vi "_Validate Lens Property.vi"(6 "Lens Property In":T8={"Scan Type"=0, "Unit"=TRUE, "Count1"=1.0, "Count2"=1.0, "Time1"=1.0, "Time2"=1.0, "Scans"=1, "Step Size"=1.0, "Row Numer"=0} {"Scan Type" items=["Single", "Dual", "Ramp"]}, 8 "Method In":T1={"Lenses"=[], "Mass Ranges"=[], "Acquire"=FALSE, "MCA"=FALSE, "Q1DC EN"=FALSE, "Q1 POL"=FALSE, "Q3 POL"=FALSE, "Q1 RF  EN"=FALSE, "Averaging"=FALSE, "Log Scale"=FALSE, "CPS"=FALSE, "Unit"=FALSE, "Data Path"=path "", "Run Mode"=enum."MRM (Q1/Q2)", "Fixed Mass (amu)"=1.0, "Q3DC EN"=FALSE, "Q3 RF  EN"=FALSE, "Negative"=FALSE} {"Mass Ranges"."Res" items=["High/High", "Medium/Medium", "Low/Low", "High/Medium", "High/Low", "Medium/High", "Medium/Low", "Low/High", "Low/Medium"]}) -> (0 "Lens Table":string[][](table), 1 "Lens Property Out":T7={"Scan Type"=0, "Unit"=TRUE, "Count1"=1.0, "Count2"=1.0, "Time1"=1.0, "Time2"=1.0, "Scans"=1, "Step Size"=1.0, "Start DAC"=1, "Ramp Time (ms)"=1} {"Scan Type" items=["Single", "Dual", "Ramp"]}, 3 "Method Out":T1={"Lenses"=[], "Mass Ranges"=[], "Acquire"=FALSE, "MCA"=FALSE, "Q1DC EN"=FALSE, "Q1 POL"=FALSE, "Q3 POL"=FALSE, "Q1 RF  EN"=FALSE, "Averaging"=FALSE, "Log Scale"=FALSE, "CPS"=FALSE, "Unit"=FALSE, "Data Path"=path "", "Run Mode"=enum."MRM (Q1/Q2)", "Fixed Mass (amu)"=1.0, "Q3DC EN"=FALSE, "Q3 RF  EN"=FALSE, "Negative"=FALSE} {"Mass Ranges"."Res" items=["High/High", "Medium/Medium", "Low/Low", "High/Medium", "High/Low", "Medium/High", "Medium/Low", "Low/High", "Low/Medium"]})   [LabVIEW 2012]
uses:
  Type/_GUI Method.ctl
  Type/_Lens Property.ctl
  Type/_Mass Range Property.ctl
  Type/_Mass Range Parameters.ctl
  Type/_RT Res Type.ctl
  Type/_Run Mode.ctl
  _Global Configuration.vi
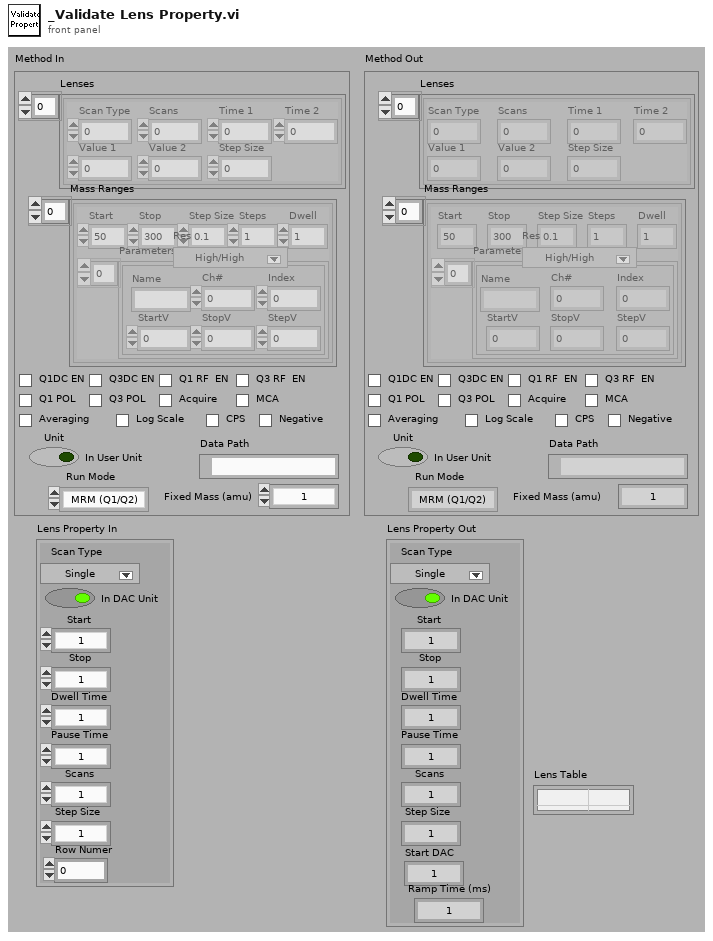
[diagram p1: front panel]
types:
  T1 = typedef "_GUI Method.ctl" = cluster{"Lenses":T2[], "Mass Ranges":T3[], "Acquire":bool, "MCA":bool, "Q1DC EN":bool, "Q1 POL":bool, "Q3 POL":bool, "Q1 RF  EN":bool, "Averaging":bool, "Log Scale":bool, "CPS":bool, "Unit":bool, "Data Path":path, "Run Mode":T6, "Fixed Mass (amu)":dbl, "Q3DC EN":bool, "Q3 RF  EN":bool, "Negative":bool}
  T2 = typedef "_Lens Property.ctl" = cluster{"Scan Type":u8, "Scans":i32, "Time 1":dbl, "Time 2":dbl, "Value 1":dbl, "Value 2":dbl, "Step Size":dbl}
  T3 = typedef "_Mass Range Property.ctl" = cluster{"Start":dbl, "Stop":dbl, "Step Size":dbl, "Steps":i32, "Dwell":dbl, "Parameters":T4[], "Res":T5}
  T4 = typedef "_Mass Range Parameters.ctl" = cluster{"Name":string, "Ch#":u8, "StartV":dbl, "StopV":dbl, "StepV":dbl, "Index":u8}
  T5 = typedef "_RT Res Type.ctl" = u16
  T6 = typedef "_Run Mode.ctl" = enum16{"MRM (Q1/Q2)", "Q1 Scan", "Q1 SRM", "Q2 Scan", "Q2 SRM", "Product Scan", "Precursor Scan", "Neutral Loss", "Neutral Gain"}
  T7 = cluster{"Scan Type":u8, "Unit":bool, "Count1":dbl, "Count2":dbl, "Time1":dbl, "Time2":dbl, "Scans":i32, "Step Size":dbl, "Start DAC":i32, "Ramp Time (ms)":i32}
  T8 = cluster{"Scan Type":u8, "Unit":bool, "Count1":dbl, "Count2":dbl, "Time1":dbl, "Time2":dbl, "Scans":i32, "Step Size":dbl, "Row Numer":i32}
  T9 = typedef "_RT Instrument 2.ctl" = cluster{"Table":T10[], "Instrument":string[]}
  T10 = typedef "_RT Configuration 2.ctl" = cluster{"Name":string, "Ch#":u8, "Min":dbl, "Max":dbl, "Def+":dbl, "Def-":dbl, "Offset":dbl, "Slope":dbl, "Type":u8, "Description":string, "SettleT":dbl}
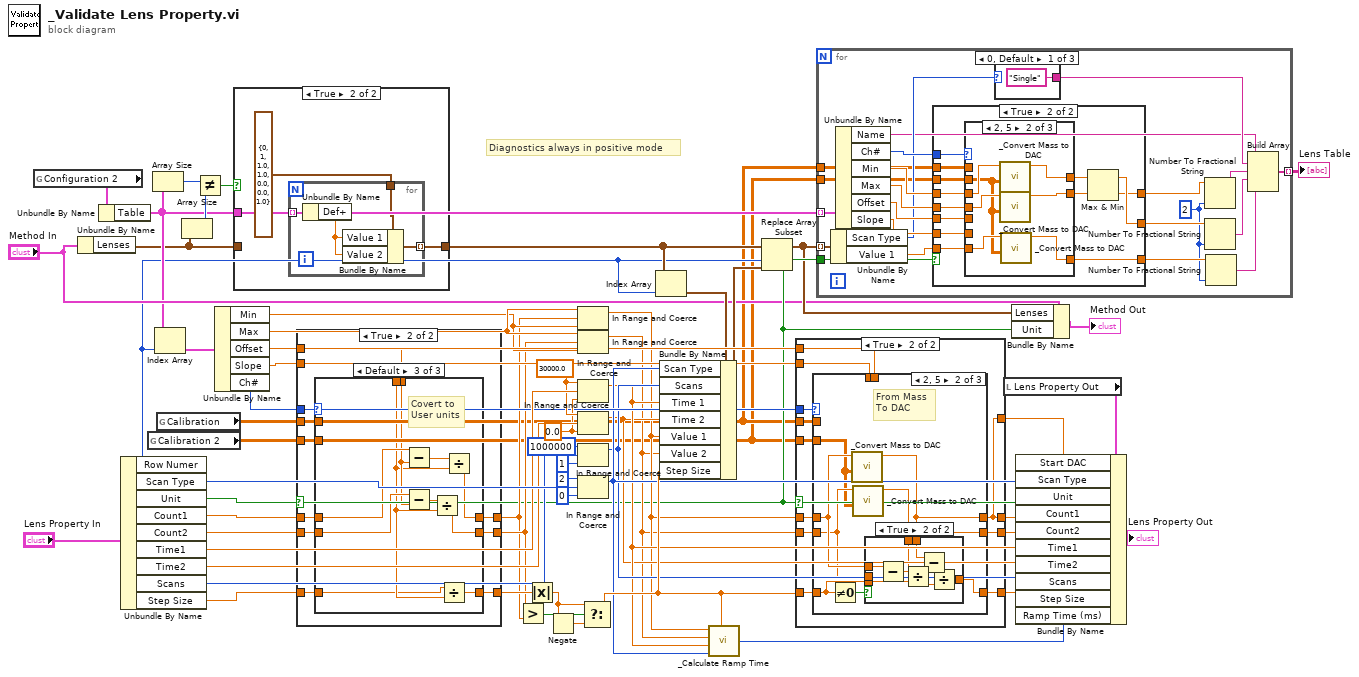
[diagram p0: block diagram]
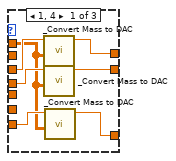
[diagram p4: hidden frame]
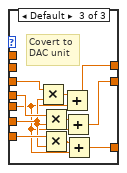
[diagram p5: hidden frame]
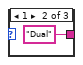
[diagram p6: hidden frame]
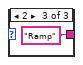
[diagram p7: hidden frame]
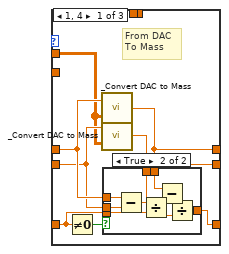
[diagram p9: hidden frame]
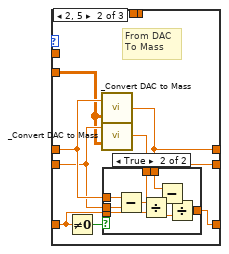
[diagram p11: hidden frame]
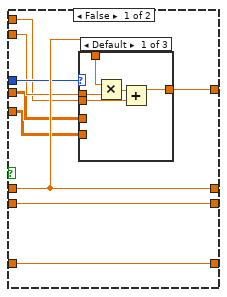
[diagram p13: hidden frame]
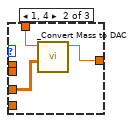
[diagram p14: hidden frame]
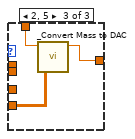
[diagram p15: hidden frame]
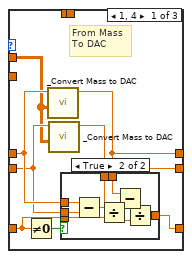
[diagram p16: hidden frame]
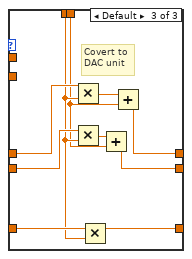
[diagram p19: hidden frame]
diagram:
  w41 = 0.0 ("lower limit")
  w43 = 30000.0 ("upper limit")
  # "Diagnostics always in positive mode"
  n1 = global read "_Global Configuration.vi" "Configuration 2"() -> (w26:T9)
  n2 = Unbundle By Name("Method In") -> ("Lenses"=w8:T2[])
  n3 = Unbundle By Name(w26) -> ("Table"=w9:T10[])
  n4 = Unbundle By Name("Lens Property In") -> ("Row Numer"=w6:i32, "Scan Type"=w57:u8, "Unit"=w16:bool, "Count1"=w56:dbl, "Count2"=w55:dbl, "Time1"=w54:dbl, "Time2"=w53:dbl, "Scans"=w52:i32, "Step Size"=w51:dbl)
  n5 = global read "_Global Configuration.vi" "Calibration 2"() -> (w1:dbl[][])
  n6 = Array Size(array=w9) -> (size(s)=w12:i32)
  n7 = Index Array(array=w9, index=w6) -> (element=w25:T10)
  n8 = global read "_Global Configuration.vi" "Calibration"() -> (w2:dbl[][])
  n9 = Array Size(array=w8) -> (size(s)=w13:i32)
  n10 = Not Equal?(x=w12, y=w13) -> (x != y?=w11:bool)
  n11 = Unbundle By Name(w25) -> ("Min"=w37:dbl, "Max"=w38:dbl, "Offset"=w39:dbl, "Slope"=w50:dbl, "Ch#"=w34:u8)
  n12 = case shown="True" w11 {
    tunnel: w9 -> [_ w61]
    tunnel: w8 -> [w58 _]
    tunnel: [w58 w59] -> w7
    frame False {
    }
    frame True {
      n13 = for {
        tunnel: w61 -> [w64] mode=indexing
        tunnel: T2 {"Scan Type"=0, "Scans"=1, "Time 1"=1.0, "Time 2"=1.0, "Value 1"=0.0, "Value 2"=0.0, "Step Size"=1.0} ("Lenses") -> [w65]
        tunnel: [w62] -> w59 mode=indexing
        n14 = Unbundle By Name(w64) -> ("Def+"=w63:dbl)
        n15 = Bundle By Name(cluster=w65, "Value 1"=w63, "Value 2"=w63) -> (w62:T2)
      }
    }
  }
  n16 = case shown="True" w16 {
    tunnel: w56 -> [w68 w79]
    tunnel: w55 -> [w67 w77]
    tunnel: [w68 w78] -> w31
    tunnel: [w67 w76] -> w32
    tunnel: w39 -> [_ w74]
    tunnel: w50 -> [_ w73]
    tunnel: [w66 w75] -> w33
    tunnel: w51 -> [w66 w72]
    tunnel: w34 -> [_ w71]
    tunnel: w2 -> [_ w70]
    tunnel: w1 -> [_ w69]
    frame False {
    }
    frame True {
      n17 = case shown="Default" w71 {
        tunnel: w79 -> [w85 w103 w125]
        tunnel: [w83 w101 w123] -> w78
        tunnel: w77 -> [w84 w102 w121]
        tunnel: [w82 w100 w120] -> w76
        tunnel: [w81 w99 w119] -> w75
        tunnel: w74 -> [_ _ w118]
        tunnel: w73 -> [_ _ w117]
        tunnel: w72 -> [w86 w104 w116]
        tunnel: w70 -> [w80 _ _]
        tunnel: w69 -> [_ w98 _]
        frame 1, 4 {
          # "From DAC\nTo Mass"
          n18 = Not Equal To 0?(x=w86) -> (x != 0?=w87:bool)
          n19 = call "_Convert DAC to Mass.vi"("Calibration Table"=w80, "DAC"=w85) -> ("Mass"=w83:dbl)
          n20 = call "_Convert DAC to Mass.vi"("Calibration Table"=w80, "DAC"=w84) -> ("Mass"=w82:dbl)
          n21 = case shown="True" w87 {
            tunnel: w86 -> [w88 w94]
            tunnel: w85 -> [_ w93]
            tunnel: w84 -> [_ w92]
            tunnel: w83 -> [_ w91]
            tunnel: w82 -> [_ w90]
            tunnel: [w88 w89] -> w81
            frame False {
            }
            frame True {
              n22 = Subtract(x=w93, y=w92) -> (x-y=w95:dbl)
              n23 = Divide(x=w95, y=w94) -> (x/y=w97:dbl)
              n24 = Subtract(x=w91, y=w90) -> (x-y=w96:dbl)
              n25 = Divide(x=w96, y=w97) -> (x/y=w89:dbl)
            }
          }
        }
        frame 2, 5 {
          # "From DAC\nTo Mass"
          n26 = Not Equal To 0?(x=w104) -> (x != 0?=w105:bool)
          n27 = call "_Convert DAC to Mass.vi"("Calibration Table"=w98, "DAC"=w103) -> ("Mass"=w101:dbl)
          n28 = call "_Convert DAC to Mass.vi"("Calibration Table"=w98, "DAC"=w102) -> ("Mass"=w100:dbl)
          n29 = case shown="True" w105 {
            tunnel: w104 -> [w106 w112]
            tunnel: w103 -> [_ w111]
            tunnel: w102 -> [_ w110]
            tunnel: w101 -> [_ w109]
            tunnel: w100 -> [_ w108]
            tunnel: [w106 w107] -> w99
            frame False {
            }
            frame True {
              n30 = Subtract(x=w111, y=w110) -> (x-y=w113:dbl)
              n31 = Divide(x=w113, y=w112) -> (x/y=w115:dbl)
              n32 = Subtract(x=w109, y=w108) -> (x-y=w114:dbl)
              n33 = Divide(x=w114, y=w115) -> (x/y=w107:dbl)
            }
          }
        }
        frame Default {
          # "Covert to\nUser units"
          n34 = Subtract(x=w125, y=w118) -> (x-y=w124:dbl)
          n35 = Subtract(x=w121, y=w118) -> (x-y=w122:dbl)
          n36 = Divide(x=w122, y=w117) -> (x/y=w120:dbl)
          n37 = Divide(x=w116, y=w117) -> (x/y=w119:dbl)
          n38 = Divide(x=w124, y=w117) -> (x/y=w123:dbl)
        }
      }
    }
  }
  n39 = Greater?(x=w32, y=w31) -> (0:w30:bool)
  n40 = Absolute Value(x=w33) -> (abs(x)=w28:dbl)
  n41 = Negate(x=w28) -> (-x=w29:dbl)
  n42 = In Range and Coerce(upper limit=w38, x=w31, lower limit=w37) -> (coerced(x)=w18:dbl)  [unwired: 1 out]
  n43 = In Range and Coerce(upper limit=w38, x=w32, lower limit=w37) -> (coerced(x)=w17:dbl)  [unwired: 1 out]
  n44 = In Range and Coerce(upper limit=w43, x=w54, lower limit=w41) -> (coerced(x)=w20:dbl)  [unwired: 1 out]
  n45 = In Range and Coerce(upper limit=w43, x=w53, lower limit=w41) -> (coerced(x)=w19:dbl)  [unwired: 1 out]
  n46 = In Range and Coerce(upper limit=1000000, x=w52, lower limit=1) -> (coerced(x)=w21:i32)  [unwired: 1 out]
  n47 = In Range and Coerce(upper limit=u8 2, x=w57, lower limit=u8 0) -> (coerced(x)=w22:u8)  [unwired: 1 out]
  n48 = Select(t=w28, s=w30, f=w29) -> (s? t:f=w27:dbl)
  n49 = Index Array(array=w7, index=w6) -> (element=w24:T2)
  n50 = Bundle By Name(cluster=w24, "Scan Type"=w22, "Scans"=w21, "Time 1"=w20, "Time 2"=w19, "Value 1"=w18, "Value 2"=w17, "Step Size"=w27) -> (w23:T2)
  n51 = call "_Calculate Ramp Time.vi"("Start"=w18, "Stop"=w17, "Dwell (ms)"=w20, "Scan Type"=w22, "Step"=w27) -> ("Ramp Time (ms)"=w3:i32)
  n52 = Replace Array Subset(array=w7, new element=w23, index=w6) -> (w15:T2[])
  n53 = case shown="True" w16 {
    tunnel: w18 -> [w132 w156]
    tunnel: w17 -> [w134 w155]
    tunnel: [w132 w148] -> w48
    tunnel: [w134 w154] -> w46
    tunnel: w39 -> [w129 w151]
    tunnel: w50 -> [w130 w152]
    tunnel: [w133 w150] -> w47
    tunnel: w27 -> [w133 w153]
    tunnel: w34 -> [w131 w149]
    tunnel: [w128 w148] -> w4
    tunnel: w2 -> [w127 w147]
    tunnel: w1 -> [w126 w146]
    frame False {
      n54 = case shown="Default" w131 {
        tunnel: w132 -> [w138 w142 w145]
        tunnel: [w135 w141 w144] -> w128
        tunnel: w130 -> [w137 _ _]
        tunnel: w129 -> [w136 _ _]
        tunnel: w127 -> [_ w140 _]
        tunnel: w126 -> [_ _ w143]
        frame Default {
          n55 = Multiply(x=w138, y=w137) -> (x*y=w139:dbl)
          n56 = Add(x=w139, y=w136) -> (x+y=w135:dbl)
        }
        frame 1, 4 {
          n57 = call "_Convert Mass to DAC.vi"("Calibration Table"=w140, "Mass"=w142) -> ("DAC Value"=w141:dbl)  [unwired: 2 in, 3 out]
        }
        frame 2, 5 {
          n58 = call "_Convert Mass to DAC.vi"("Calibration Table"=w143, "Mass"=w145) -> ("DAC Value"=w144:dbl)  [unwired: 2 in, 3 out]
        }
      }
    }
    frame True {
      n59 = case shown="2, 5" w149 {
        tunnel: w156 -> [w162 w180 w202]
        tunnel: [w158 w176 w200] -> w148
        tunnel: w155 -> [w161 w179 w198]
        tunnel: [w159 w177 w197] -> w154
        tunnel: w153 -> [w160 w178 w196]
        tunnel: w152 -> [_ _ w195]
        tunnel: w151 -> [_ _ w194]
        tunnel: [w164 w182 w193] -> w150
        tunnel: w147 -> [w157 _ _]
        tunnel: w146 -> [_ w175 _]
        frame 1, 4 {
          # "From Mass\nTo DAC"
          n60 = Not Equal To 0?(x=w160) -> (x != 0?=w163:bool)
          n61 = call "_Convert Mass to DAC.vi"("Calibration Table"=w157, "Mass"=w162) -> ("DAC Value"=w158:dbl)  [unwired: 2 in, 3 out]
          n62 = call "_Convert Mass to DAC.vi"("Calibration Table"=w157, "Mass"=w161) -> ("DAC Value"=w159:dbl)  [unwired: 2 in, 3 out]
          n63 = case shown="True" w163 {
            tunnel: w160 -> [w165 w171]
            tunnel: w162 -> [_ w170]
            tunnel: w161 -> [_ w169]
            tunnel: w158 -> [_ w168]
            tunnel: w159 -> [_ w167]
            tunnel: [w165 w166] -> w164
            frame False {
            }
            frame True {
              n64 = Subtract(x=w170, y=w169) -> (x-y=w172:dbl)
              n65 = Divide(x=w172, y=w171) -> (x/y=w174:dbl)
              n66 = Subtract(x=w168, y=w167) -> (x-y=w173:dbl)
              n67 = Divide(x=w173, y=w174) -> (x/y=w166:dbl)
            }
          }
        }
        frame 2, 5 {
          # "From Mass\nTo DAC"
          n68 = Not Equal To 0?(x=w178) -> (x != 0?=w181:bool)
          n69 = call "_Convert Mass to DAC.vi"("Calibration Table"=w175, "Mass"=w180) -> ("DAC Value"=w176:dbl)  [unwired: 2 in, 3 out]
          n70 = call "_Convert Mass to DAC.vi"("Calibration Table"=w175, "Mass"=w179) -> ("DAC Value"=w177:dbl)  [unwired: 2 in, 3 out]
          n71 = case shown="True" w181 {
            tunnel: w178 -> [w183 w189]
            tunnel: w180 -> [_ w188]
            tunnel: w179 -> [_ w187]
            tunnel: w176 -> [_ w186]
            tunnel: w177 -> [_ w185]
            tunnel: [w183 w184] -> w182
            frame False {
            }
            frame True {
              n72 = Subtract(x=w188, y=w187) -> (x-y=w190:dbl)
              n73 = Divide(x=w190, y=w189) -> (x/y=w192:dbl)
              n74 = Subtract(x=w186, y=w185) -> (x-y=w191:dbl)
              n75 = Divide(x=w191, y=w192) -> (x/y=w184:dbl)
            }
          }
        }
        frame Default {
          # "Covert to\nDAC unit"
          n76 = Multiply(x=w202, y=w195) -> (x*y=w201:dbl)
          n77 = Multiply(x=w198, y=w195) -> (x*y=w199:dbl)
          n78 = Multiply(x=w196, y=w195) -> (x*y=w193:dbl)
          n79 = Add(x=w199, y=w194) -> (x+y=w197:dbl)
          n80 = Add(x=w201, y=w194) -> (x+y=w200:dbl)
        }
      }
    }
  }
  n81 = for {
    tunnel: w15 -> [w211] mode=indexing
    tunnel: w16 -> [w224]
    tunnel: [w217] -> w36 mode=indexing
    tunnel: w9 -> [w212] mode=indexing
    tunnel: w2 -> [w204]
    tunnel: w1 -> [w203]
    w208 = 2
    n82 = Unbundle By Name(w211) -> ("Scan Type"=w209:u8, "Value 1"=w210:dbl)
    n83 = Unbundle By Name(w212) -> ("Name"=w205:string, "Ch#"=w213:u8, "Min"=w219:dbl, "Max"=w221:dbl, "Offset"=w223:dbl, "Slope"=w222:dbl)
    n84 = case shown="True" w224 {
      tunnel: w223 -> [_ w232]
      tunnel: w222 -> [_ w233]
      tunnel: w219 -> [w227 w240]
      tunnel: w221 -> [w226 w239]
      tunnel: [w227 w235] -> w218
      tunnel: [w226 w236] -> w220
      tunnel: [w225 w231] -> w215
      tunnel: w210 -> [w225 w234]
      tunnel: w213 -> [_ w230]
      tunnel: w204 -> [_ w229]
      tunnel: w203 -> [_ w228]
      frame False {
      }
      frame True {
        n85 = case shown="2, 5" w230 {
          tunnel: w240 -> [w247 w254 w263]
          tunnel: w239 -> [w246 w253 w262]
          tunnel: [w245 w252 w261] -> w238
          tunnel: [w244 w251 w260] -> w237
          tunnel: w234 -> [w243 w250 w258]
          tunnel: w233 -> [_ _ w257]
          tunnel: w232 -> [_ _ w256]
          tunnel: [w242 w249 w255] -> w231
          tunnel: w229 -> [w241 _ _]
          tunnel: w228 -> [_ w248 _]
          frame 1, 4 {
            n86 = call "_Convert Mass to DAC.vi"("Calibration Table"=w241, "Mass"=w247) -> ("DAC Value"=w245:dbl)  [unwired: 2 in, 3 out]
            n87 = call "_Convert Mass to DAC.vi"("Calibration Table"=w241, "Mass"=w246) -> ("DAC Value"=w244:dbl)  [unwired: 2 in, 3 out]
            n88 = call "_Convert Mass to DAC.vi"("Calibration Table"=w241, "Mass"=w243) -> ("DAC Value"=w242:dbl)  [unwired: 2 in, 3 out]
          }
          frame 2, 5 {
            n89 = call "_Convert Mass to DAC.vi"("Calibration Table"=w248, "Mass"=w254) -> ("DAC Value"=w252:dbl)  [unwired: 2 in, 3 out]
            n90 = call "_Convert Mass to DAC.vi"("Calibration Table"=w248, "Mass"=w253) -> ("DAC Value"=w251:dbl)  [unwired: 2 in, 3 out]
            n91 = call "_Convert Mass to DAC.vi"("Calibration Table"=w248, "Mass"=w250) -> ("DAC Value"=w249:dbl)  [unwired: 2 in, 3 out]
          }
          frame Default {
            # "Covert to\nDAC unit"
            n92 = Multiply(x=w263, y=w257) -> (x*y=w265:dbl)
            n93 = Multiply(x=w262, y=w257) -> (x*y=w264:dbl)
            n94 = Multiply(x=w258, y=w257) -> (x*y=w259:dbl)
            n95 = Add(x=w265, y=w256) -> (x+y=w261:dbl)
            n96 = Add(x=w264, y=w256) -> (x+y=w260:dbl)
            n97 = Add(x=w259, y=w256) -> (x+y=w255:dbl)
          }
        }
        n98 = Max & Min(x=w238, y=w237) -> (max(x,y)=w236:dbl, min(x,y)=w235:dbl)
      }
    }
    n99 = case shown="0, Default" w209 {
      tunnel: ["Single" ("Scan Type") "Dual" ("Scan Type") "Ramp" ("Scan Type")] -> w207
      frame 0, Default {
      }
      frame 1 {
      }
      frame 2 {
      }
    }
    n100 = Number To Fractional String(number=w218, precision (6)=w208) -> (F-format string=w206:string)  [unwired: 2 out]
    n101 = Number To Fractional String(number=w220, precision (6)=w208) -> (F-format string=w216:string)  [unwired: 2 out]
    n102 = Number To Fractional String(number=w215, precision (6)=w208) -> (F-format string=w214:string)  [unwired: 2 out]
    n103 = Build Array(w205, w207, w206, w216, w214) -> (w217:string[])
  }
  "Lens Table" <- w36
  n104 = local read "Lens Property Out"() -> (w5:T7)
  n105 = Bundle By Name(cluster="Method In", "Lenses"=w15, "Unit"=w16) -> (→"Method Out":T1)
  n106 = Bundle By Name(cluster=w5, "Start DAC"=w4, "Scan Type"=w22, "Unit"=w16, "Count1"=w48, "Count2"=w46, "Time1"=w20, "Time2"=w19, "Scans"=w21, "Step Size"=w47, "Ramp Time (ms)"=w3) -> (→"Lens Property Out":T7)
